vi "Canceled.vi"(8 "error in (no error)":errorcluster, 9 "Timeout (0)":i32, 11 "UI Events Registration":refnum<event-registration>) -> (0 "error out":errorcluster, 2 "Canceled by user?":bool)   [LabVIEW 2015, in "Simple Progress Bar.lvlib"]
uses:
  Simple Progress Bar.lvlib
  UI Events.ctl
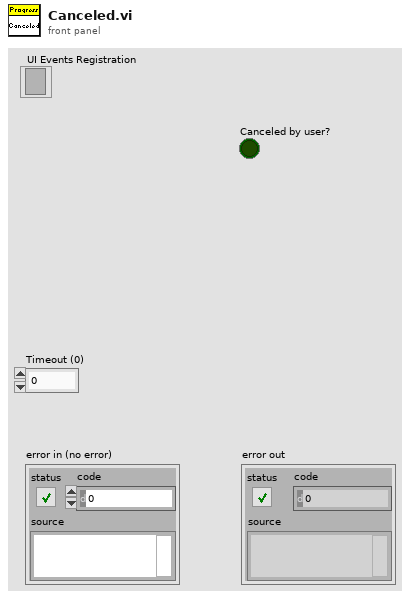
[diagram p1: front panel]
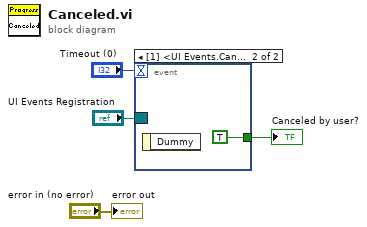
[diagram p0: block diagram]
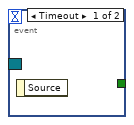
[diagram p2: hidden frame]
diagram:
  n1 = event shown="[1] <UI Events.Cancel>: User Event" {
    selector: "UI Events Registration" -> [_ _]
    dyn-events: _ -> [_ _]
    timeout: "Timeout (0)" -> [_ _]
    tunnel: [_ TRUE] -> w3
    event Timeout {
      n2 = event-data() -> ()  [unwired: 1 in, 1 out]
    }
    event User Event {
      n3 = event-data() -> ()  [unwired: 1 in, 1 out]
    }
  }
  "Canceled by user?" <- w3
  "error out" <- "error in (no error)"
